vi "Library VI dependent on missing VI.vi"   [LabVIEW 2023, in "Library.lvlib"]
uses:
  Library.lvlib
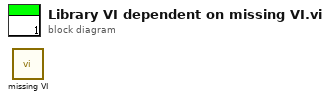
[diagram p0: block diagram]
diagram:
  n1 = call "missing VI.vi"() -> ()  [unwired: 12 in]
